vi "Data.Write Data to HW.vi"(8 "error in (no error)":errorcluster, 11 "Data Access API in":refnum<class "Data Access API.lvclass">) -> (0 "error out":errorcluster, 3 "Data Access API out":refnum<class "Data Access API.lvclass">)   [LabVIEW 2015, in "Data Access API.lvlib" / "Data Access API.lvclass"]
uses:
  Data Access API.lvclass
  Data Access API.lvclass/Data Access API.ctl
  Data/Read/Read.lvclass/Read.ctl
  <vilib>/NI Veristand/Custom Device API/NI VeriStand - Get Channel Values by Block Data Reference.vi
  <vilib>/NI Veristand/Custom Device API/Global Data Refs.vi
  Data/Read/Read.lvclass
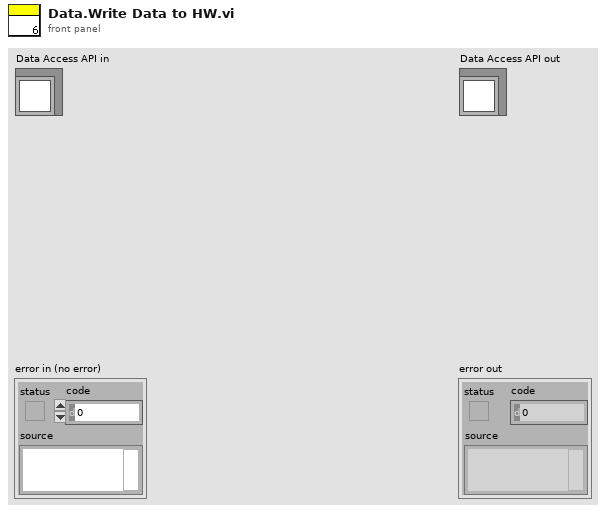
[diagram p1: front panel]
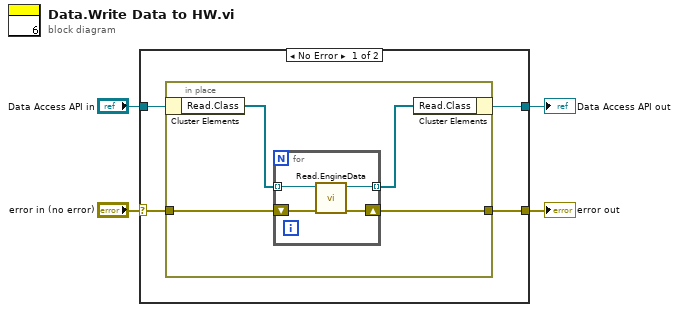
[diagram p0: block diagram]
diagram:
  n1 = case shown="No Error" "error in (no error)" {
    selector: "error in (no error)" -> [w6 w18]
    tunnel: [w8 w18] -> w3
    tunnel: [w7 w17] -> w1
    tunnel: "Data Access API in" -> [w5 w17]
    frame No Error {
      n2 = in-place {
        in-place-border: w6 -> [w9]
        in-place-border: [w12] -> w8
        n3 = in-place-cluster #1(w5) -> ("Read.Class"=w11:refnum<class "Read.lvclass">[])
        n4 = for {
          tunnel: w11 -> [w15] mode=indexing
          shift-right: [w14] -> w12
          shift-left: w9 -> [w16]
          tunnel: [w13] -> w10 mode=indexing
          n5 = call "Read.EngineData.vi"("error in"=w16, "Read in"=w15) -> ("error out"=w14:errorcluster, "Read out"=w13:refnum<class "Read.lvclass">)  [unwired: 8 in]
        }
        n6 = in-place-cluster #1("Read.Class"=w10) -> (w7:refnum<class "Data Access API.lvclass">)
      }
    }
    frame Error {
    }
  }
  "error out" <- w3
  "Data Access API out" <- w1
